vi "tcp.vi"   [LabVIEW 2020]
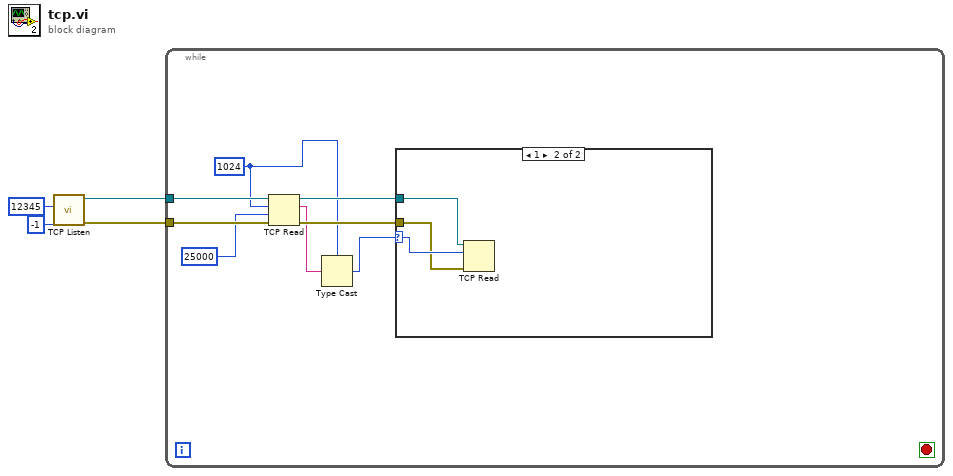
[diagram p0: block diagram]
diagram:
  n1 = call <vilib>:"TCP Listen.vi"("timeout ms (wait forever: -1)"=-1, "port"=u16 12345) -> ("error out"=w1:errorcluster, "connection ID"=w2:refnum<k5>)  [unwired: 5 in, 3 out]
  n2 = while {
    tunnel: w2 -> [w12]
    tunnel: w1 -> [w11]
    stop <- _ stop-if-true
    w7 = 1024 ("bytes to read")
    n3 = TCP Read(connection ID=w12, bytes to read=w7, error in (no error)=w11, 9:25000 ("timeout ms (25000)")) -> (connection ID out=w9:refnum<k5>, data out=w6:string, error out=w8:errorcluster)  [unwired: 1 in]
    n4 = Type Cast(type=w7, x=w6) -> (*(type *) &x=w5:i32)
    n5 = case shown="1" w5 {
      selector: w5 -> [_ w15]
      tunnel: w9 -> [_ w14]
      tunnel: w8 -> [_ w13]
      frame 0, Default {
      }
      frame 1 {
        n6 = TCP Read(connection ID=w14, bytes to read=w15, error in (no error)=w13) -> ()  [unwired: 2 in, 3 out]
      }
    }
  }
